vi "File Stuff.vi"() -> ()   [LabVIEW 2013]
panel:
  out "file or folder exists?":bool
  in  "error in":errorcluster
  out "path out":path
  out "error out 2":errorcluster
  out "folder names":string[](array[string])
  out "free (bytes)":i64
  out "error out":errorcluster
  in  "path":path
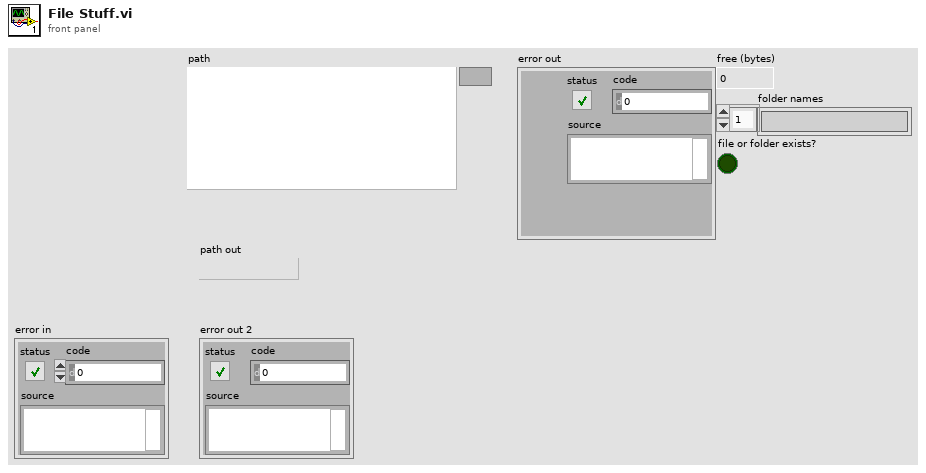
[diagram p1: front panel]
types:
  T1 = typedef "LVDateTimeRec.ctl" = cluster{"fractional second":dbl, "second":i32, "minute":i32, "hour":i32, "day of month":i32, "month":i32, "year":i32, "day of week":i32, "day of year":i32, "DST":i32}
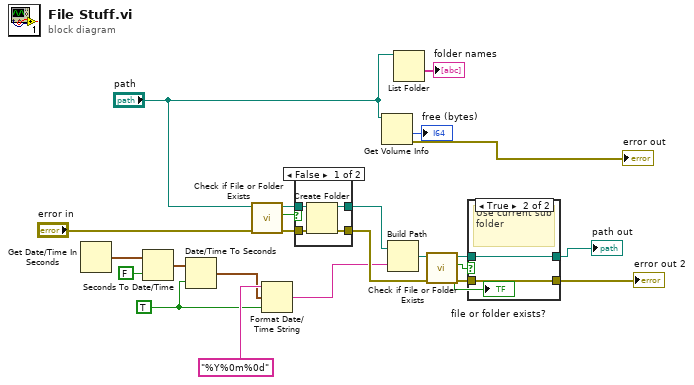
[diagram p0: block diagram]
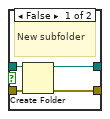
[diagram p3: hidden frame]
diagram:
  w9 = TRUE ("is UTC (F)")
  n1 = Get Date/Time In Seconds() -> (seconds since 1Jan1904=w6:timestamp)
  n2 = Seconds To Date/Time(time stamp (now)=w6, to UTC (F)=FALSE) -> (date time rec=w8:T1)
  n3 = Date/Time To Seconds(1:w9, 2:w8) -> (0:w16:timestamp)
  n4 = call <vilib>:"Check if File or Folder Exists.vi"("error in (no error)"="error in", "path"="path") -> ("error out"=w12:errorcluster, "file or folder exists?"=w20:bool, "dup path"=w11:path)  [unwired: 7 in]
  n5 = Format Date/Time String(time format string (%c)="%Y%0m%0d", seconds (now)=w16, UTC format=w9) -> (date/time string=w10:string)
  n6 = case shown="False" w20 {
    tunnel: w11 -> [w27 w29]
    tunnel: w12 -> [w26 w28]
    tunnel: [w25 w29] -> w13
    tunnel: [w24 w28] -> w14
    frame False {
      n7 = Create Folder(path (use dialog)=w27, error in=w26) -> (created path=w25:path, error out=w24:errorcluster)  [unwired: 1 in, 1 out]
    }
    frame True {
    }
  }
  n8 = Get Volume Info(11:"path") -> (0:→"error out":errorcluster, 1:→"free (bytes)":i64)  [unwired: 1 in, 4 out]
  n9 = Build Path(base path=w13, name or relative path=w10) -> (appended path=w5:path)
  n10 = List Folder(path="path") -> (folder names=→"folder names":string[])  [unwired: 3 in, 3 out]
  n11 = call <vilib>:"Check if File or Folder Exists.vi"("error in (no error)"=w14, "path"=w5) -> ("error out"=w2:errorcluster, "file or folder exists?"=w4:bool, "dup path"=w3:path)  [unwired: 7 in]
  "file or folder exists?" <- w4
  n12 = case "No directory with current date?\nMake one" shown="True" w4 {
    tunnel: w3 -> [w32 w35]
    tunnel: [w33 w35] -> w18
    tunnel: w2 -> [w31 w34]
    tunnel: [w30 w34] -> w19
    frame False {
      # "New subfolder"
      n13 = Create Folder(path (use dialog)=w32, error in=w31) -> (created path=w33:path, error out=w30:errorcluster)  [unwired: 1 in, 1 out]
    }
    frame True {
      # "Use current sub folder"
    }
  }
  "error out 2" <- w19
  "path out" <- w18
